vi "Move Set on Cursor Move.vi"(8 "Cursor.Position.X":dbl, 9 "Cursor Name":string, 10 "Refnums for Resizing and Alignment":T1, 11 "Display State In":T2={"Graph Visible Items"={"Plot Legend"=FALSE, "Scale Legend"=FALSE, "Graph Palette"=FALSE, "Cursor Legend"=FALSE, "X Scrollbar"=FALSE}, "View Table"=FALSE, "Table Visible Items"={"Vertical Scrollbar"=FALSE, "Horizontal Scrollbar"=FALSE, "Row Headers"=FALSE, "Column Headers"=FALSE, "Vertical Lines"=FALSE, "Horizontal Lines"=FALSE}, "Header Font"={"Font Name"="", "Size"=0, "Bold"=FALSE, "Italic"=FALSE, "Underline"=FALSE, "Strikeout"=FALSE, "Color"=0}, "Cell Font"={"Font Name"="", "Size"=0, "Bold"=FALSE, "Italic"=FALSE, "Underline"=FALSE, "Strikeout"=FALSE, "Color"=0}, "Description and Tip..."={"Description"="", "Tip"=""}, "Moveable Splitter Position"=0, "Measurement Cursor Configuration"={"relative to t0"={"enable relative time"=FALSE, "Relative times (DT)"=[], "color"=0}, "range"={"enable range"=FALSE, "T1"=0.0, "T2"=0.0, "Fixed interval (T2-T1)"=0.0, "T1 color"=0, "T2 color"=0, "enable shading"=FALSE}, "periodic"={"enable periodic"=FALSE, "First event (E1)"=0.0, "Number events (Ei)"=0, "Event spacing (s)"=0.0, "First color"=0, "Events color"=0}, "absolute timestamp"={"enable absolute"=FALSE, "Timestamps (TS)"=[], "color"=0}}, "X Increment"=0.0, "X Scale"={"Label Visible"=FALSE, "Label Text"="", "Time Mode"=enum."Relative", "Format String"=""}, "Y Scale"={"Label Visible"=FALSE, "Label Text"="", "Scaling"=enum."Engineering Units", "Format String"=""}, "Colors"={"background"=16777215, "major grid"=8355711, "minor grid"=12632256, "font"=0}, "Cursors"={"List"=[], "Tags"=[]}, "Plots"=[], "Plot Color Wheel"=[3381759, 32768, 982784, 4375295, 13827953, 13457919, 16757522, 4343295, 16728758, 12095254], "registered user events"=variant} caption="State") -> (1 "state changed":bool, 3 "Display State Out":T2={"Graph Visible Items"={"Plot Legend"=FALSE, "Scale Legend"=FALSE, "Graph Palette"=FALSE, "Cursor Legend"=FALSE, "X Scrollbar"=FALSE}, "View Table"=FALSE, "Table Visible Items"={"Vertical Scrollbar"=FALSE, "Horizontal Scrollbar"=FALSE, "Row Headers"=FALSE, "Column Headers"=FALSE, "Vertical Lines"=FALSE, "Horizontal Lines"=FALSE}, "Header Font"={"Font Name"="", "Size"=0, "Bold"=FALSE, "Italic"=FALSE, "Underline"=FALSE, "Strikeout"=FALSE, "Color"=0}, "Cell Font"={"Font Name"="", "Size"=0, "Bold"=FALSE, "Italic"=FALSE, "Underline"=FALSE, "Strikeout"=FALSE, "Color"=0}, "Description and Tip..."={"Description"="", "Tip"=""}, "Moveable Splitter Position"=0, "Measurement Cursor Configuration"={"relative to t0"={"enable relative time"=FALSE, "Relative times (DT)"=[], "color"=0}, "range"={"enable range"=FALSE, "T1"=0.0, "T2"=0.0, "Fixed interval (T2-T1)"=0.0, "T1 color"=0, "T2 color"=0, "enable shading"=FALSE}, "periodic"={"enable periodic"=FALSE, "First event (E1)"=0.0, "Number events (Ei)"=0, "Event spacing (s)"=0.0, "First color"=0, "Events color"=0}, "absolute timestamp"={"enable absolute"=FALSE, "Timestamps (TS)"=[], "color"=0}}, "X Increment"=0.0, "X Scale"={"Label Visible"=FALSE, "Label Text"="", "Time Mode"=enum."Relative", "Format String"=""}, "Y Scale"={"Label Visible"=FALSE, "Label Text"="", "Scaling"=enum."Engineering Units", "Format String"=""}, "Colors"={"background"=16777215, "major grid"=8355711, "minor grid"=12632256, "font"=0}, "Cursors"={"List"=[], "Tags"=[]}, "Plots"=[], "Plot Color Wheel"=[3381759, 32768, 982784, 4375295, 13827953, 13457919, 16757522, 4343295, 16728758, 12095254], "registered user events"=variant} caption="State")   [LabVIEW 2017, in "Waveforms with Cursors.xctl"]
doc: "Moves linked cursors in set. Also sets cursor selection in cursor table."
uses:
  <vilib>/addons/_XControls/Waveforms with Cursors/Waveforms with Cursors.xctl
  <vilib>/addons/_XControls/Waveforms with Cursors/Controls/State.ctl
  <vilib>/Utility/miscctls.llb/LVFontTypeDef.ctl
  <vilib>/addons/_XControls/Waveforms with Cursors/Controls/Waveform Cursor Configuration.ctl
  <vilib>/addons/_XControls/Waveforms with Cursors/Controls/Refnums Typedef.ctl
  <vilib>/Utility/miscctls.llb/LVRowAndColumnTypeDef.ctl
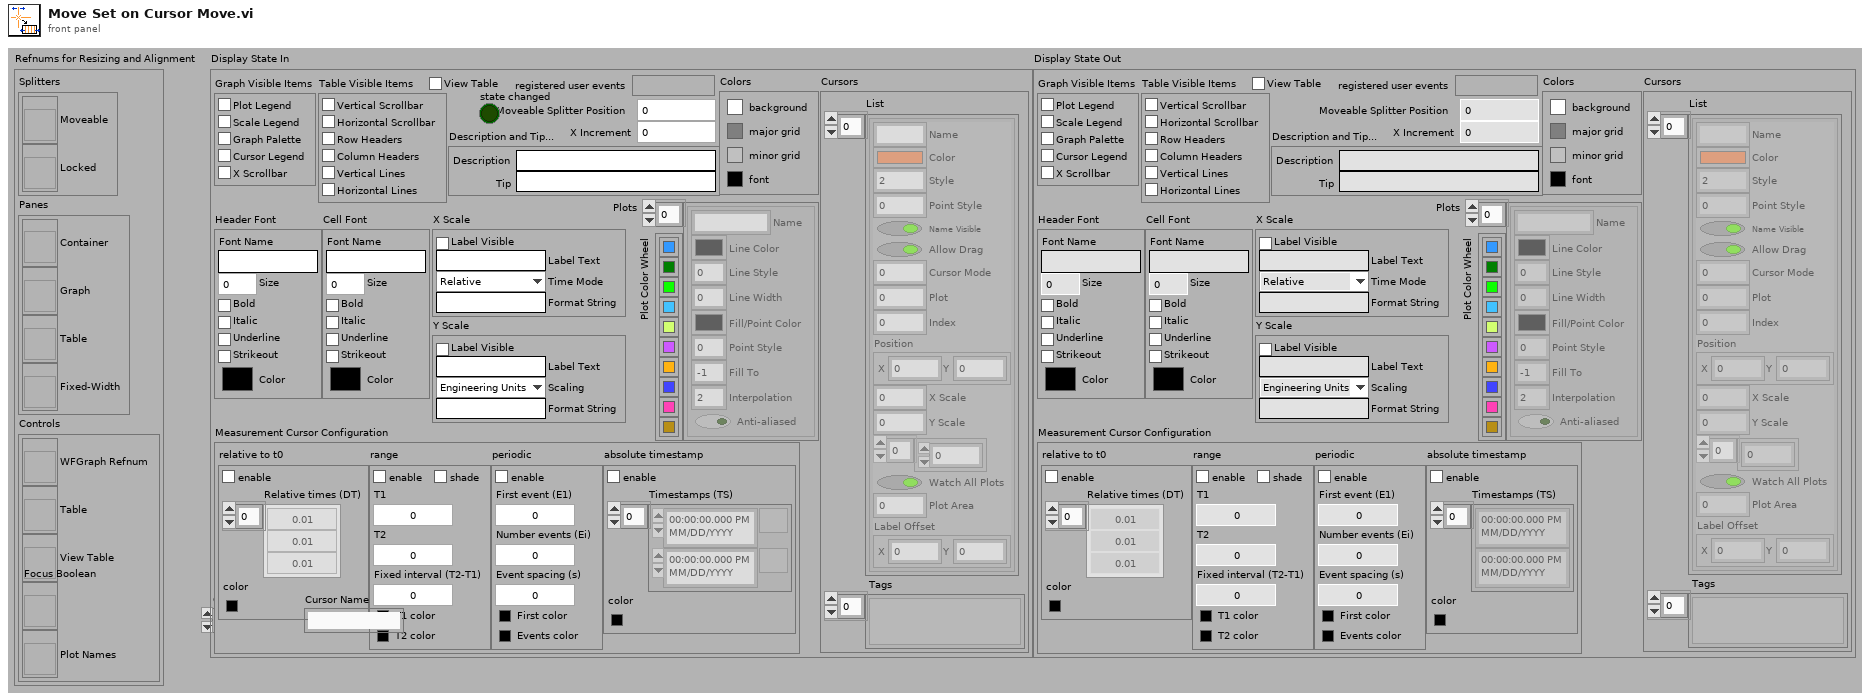
[diagram p1: front panel]
types:
  T1 = typedef "Waveforms with Cursors.xctl/Refnums Typedef.ctl" = cluster{"Splitters":cluster{"Moveable":refnum<vi>, "Locked":refnum<vi>}, "Panes":cluster{"Container":refnum<vi>, "Graph":refnum<vi>, "Table":refnum<vi>, "Fixed-Width":refnum<vi>}, "Controls":cluster{"WFGraph Refnum":refnum<vi>, "Table":refnum<vi>, "View Table":refnum<vi>, "Focus Boolean":refnum<vi>, "Plot Names":refnum<vi>}}
  T2 = typedef "Waveforms with Cursors.xctl/State.ctl" = cluster{"Graph Visible Items":cluster{"Plot Legend":bool, "Scale Legend":bool, "Graph Palette":bool, "Cursor Legend":bool, "X Scrollbar":bool}, "View Table":bool, "Table Visible Items":cluster{"Vertical Scrollbar":bool, "Horizontal Scrollbar":bool, "Row Headers":bool, "Column Headers":bool, "Vertical Lines":bool, "Horizontal Lines":bool}, "Header Font":T3, "Cell Font":T3, "Description and Tip...":cluster{"Description":string, "Tip":string}, "Moveable Splitter Position":i32, "Measurement Cursor Configuration":T4, "X Increment":dbl, "X Scale":cluster{"Label Visible":bool, "Label Text":string, "Time Mode":enum16{"Relative", "Absolute"}, "Format String":string}, "Y Scale":cluster{"Label Visible":bool, "Label Text":string, "Scaling":enum16{"Engineering Units", "Voltage"}, "Format String":string}, "Colors":cluster{"background":u32, "major grid":u32, "minor grid":u32, "font":u32}, "Cursors":cluster{"List":cluster{"Name":string, "Color":u32, "Style":i32, "Point Style":u8, "Name Visible":bool, "Allow Drag":bool, "Cursor Mode":u32, "Plot":i32, "Index":i32, "Position":cluster{"X":dbl, "Y":dbl}, "X Scale":u32, "Y Scale":u32, "Watch Plots":i32[], "Watch All Plots":bool, "Plot Area":i32, "Label Offset":cluster{"X":dbl, "Y":dbl}}[], "Tags":variant[]}, "Plots":cluster{"Name":string, "Line Color":u32, "Line Style":u8, "Line Width":u8, "Fill/Point Color":u32, "Point Style":u8, "Fill To":i16, "Interpolation":u8, "Anti-aliased":bool}[], "Plot Color Wheel":u32[], "registered user events":variant}
  T3 = typedef "LVFontTypeDef.ctl" = cluster{"Font Name":string, "Size":u16, "Bold":bool, "Italic":bool, "Underline":bool, "Strikeout":bool, "Color":u32}
  T4 = typedef "Waveforms with Cursors.xctl/Waveform Cursor Configuration.ctl" = cluster{"relative to t0":cluster{"enable relative time":bool, "Relative times (DT)":dbl[], "color":u32}, "range":cluster{"enable range":bool, "T1":dbl, "T2":dbl, "Fixed interval (T2-T1)":dbl, "T1 color":u32, "T2 color":u32, "enable shading":bool}, "periodic":cluster{"enable periodic":bool, "First event (E1)":dbl, "Number events (Ei)":i32, "Event spacing (s)":dbl, "First color":u32, "Events color":u32}, "absolute timestamp":cluster{"enable absolute":bool, "Timestamps (TS)":timestamp[], "color":u32}}
  T5 = cluster{"Name":string, "Color":u32, "Style":i32, "Point Style":u8, "Name Visible":bool, "Allow Drag":bool, "Cursor Mode":u32, "Plot":i32, "Index":i32, "Position":cluster{"X":dbl, "Y":dbl}, "X Scale":u32, "Y Scale":u32, "Watch Plots":i32[], "Watch All Plots":bool, "Plot Area":i32, "Label Offset":cluster{"X":dbl, "Y":dbl}}[]
  T6 = typedef "LVRowAndColumnTypeDef.ctl" = cluster{"Row":i32, "Column":i32}
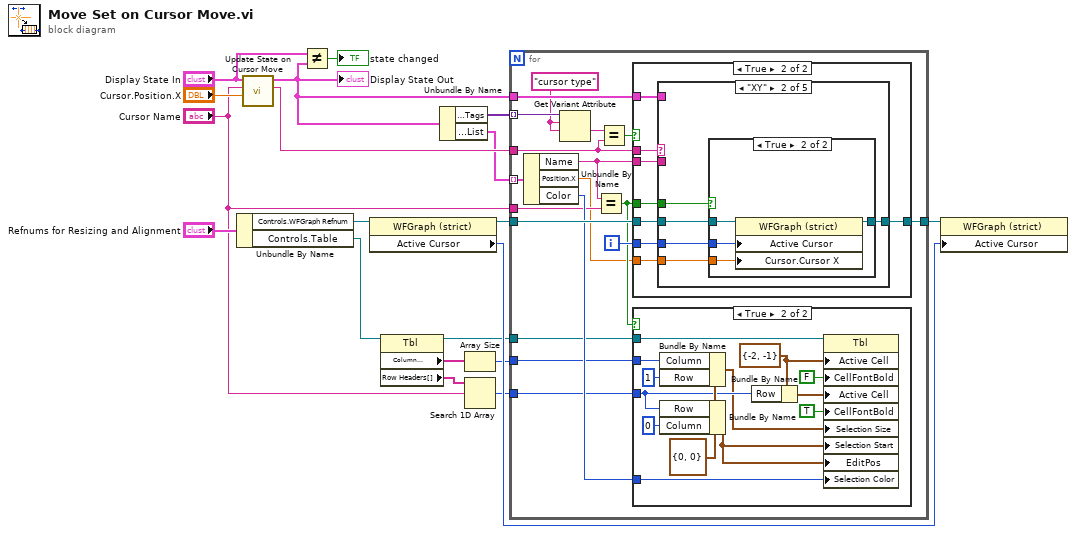
[diagram p0: block diagram]
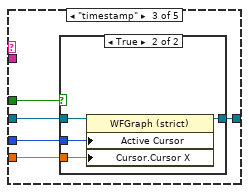
[diagram p6: hidden frame]
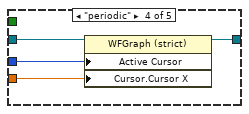
[diagram p8: hidden frame]
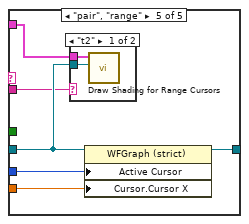
[diagram p9: hidden frame]
diagram:
  n1 = Unbundle By Name("Refnums for Resizing and Alignment") -> ("Controls.WFGraph Refnum"=w14:refnum<vi>, "Controls.Table"=w2:refnum<vi>)
  n2 = call <vilib>:"Update State on Cursor Move.vi"("Cursor.Position.X"="Cursor.Position.X", "Cursor Name"="Cursor Name", "Display State In"="Display State In") -> ("cursor type"=w12:string, "Display State out"=w10:T2)  [unwired: 7 in]
  "Display State Out" <- w10
  n3 = Not Equal?(x="Display State In", y=w10) -> (x != y?=→"state changed":bool)
  n4 = property class="WFGraph (strict)"(reference=w14) -> (reference out=w15:refnum<vi>, "Active Cursor"=w16:u32)  [unwired: 1 in, 1 out]
  n5 = property class="Tbl"(reference=w2) -> (reference out=w1:refnum<vi>, "Column Headers[]"=w6:string[], "Row Headers[]"=w7:string[])  [unwired: 1 in, 1 out]
  n6 = Unbundle By Name(w10) -> ("Cursors.Tags"=w11:variant[], "Cursors.List"=w8:T5)
  n7 = Array Size(array=w6) -> (size(s)=w5:i32)
  n8 = Search 1D Array(1D array=w7, element="Cursor Name") -> (index of element=w3:i32)  [unwired: 1 in]
  n9 = for {
    tunnel: w12 -> [w35]
    tunnel: w15 -> [w33]
    tunnel: "Cursor Name" -> [w24]
    tunnel: [w30] -> w13
    tunnel: w10 -> [w31]
    tunnel: w11 -> [w29] mode=indexing
    tunnel: w8 -> [w28] mode=indexing
    tunnel: w1 -> [w23]
    tunnel: w5 -> [w22]
    tunnel: w3 -> [w21]
    i -> [w32]
    w27 = "cursor type"
    n10 = Unbundle By Name(w28) -> ("Name"=w34:string, "Position.X"=w20:dbl, "Color"=w26:u32)
    n11 = Get Variant Attribute(Variant=w29, name=w27, default value (empty Variant)=w27) -> (value=w36:string)  [unwired: 1 in, 3 out]
    n12 = Equal?(x=w34, y=w24) -> (x = y?=w25:bool)
    n13 = Equal?(x=w36, y=w35) -> (x = y?=w37:bool)
    n14 = case shown="True" w37 {
      tunnel: w31 -> [_ w59]
      tunnel: w35 -> [_ w58]
      tunnel: w33 -> [w51 w57]
      tunnel: w25 -> [_ w54]
      tunnel: w34 -> [_ w56]
      tunnel: w32 -> [_ w55]
      tunnel: [w51 w53] -> w30
      tunnel: w20 -> [_ w52]
      frame False {
      }
      frame True {
        n15 = case shown="\"XY\"" w58 {
          tunnel: w59 -> [_ _ _ _ w88]
          tunnel: w57 -> [w60 w65 w75 w83 w87]
          tunnel: w56 -> [_ _ _ _ w85]
          tunnel: w55 -> [_ w64 w74 w84 w90]
          tunnel: w54 -> [_ w63 w73 _ _]
          tunnel: [w60 w62 w72 w82 w89] -> w53
          tunnel: w52 -> [_ w61 w71 w81 w86]
          frame Default {
          }
          frame "XY" {
            n16 = case shown="True" w63 {
              tunnel: w65 -> [w66 w70]
              tunnel: w61 -> [_ w69]
              tunnel: w64 -> [_ w68]
              tunnel: [w66 w67] -> w62
              frame False {
              }
              frame True {
                n17 = property class="WFGraph (strict)"(reference=w70, "Active Cursor"=w68, "Cursor.Cursor X"=w69) -> (reference out=w67:refnum<vi>)  [unwired: 1 in, 1 out]
              }
            }
          }
          frame "timestamp" {
            n18 = case shown="True" w73 {
              tunnel: w75 -> [w76 w80]
              tunnel: w71 -> [_ w79]
              tunnel: w74 -> [_ w78]
              tunnel: [w76 w77] -> w72
              frame False {
              }
              frame True {
                n19 = property class="WFGraph (strict)"(reference=w80, "Active Cursor"=w78, "Cursor.Cursor X"=w79) -> (reference out=w77:refnum<vi>)  [unwired: 1 in, 1 out]
              }
            }
          }
          frame "periodic" {
            n20 = property class="WFGraph (strict)"(reference=w83, "Active Cursor"=w84, "Cursor.Cursor X"=w81) -> (reference out=w82:refnum<vi>)  [unwired: 1 in, 1 out]
          }
          frame "pair", "range" {
            n21 = case shown="\"t2\"" w85 {
              tunnel: w88 -> [w92 _]
              tunnel: w87 -> [w91 _]
              frame "t2" {
                n22 = call <vilib>:"Draw Shading for Range Cursors.vi"("WaveformGraph"=w91, "Display State In"=w92) -> ()  [unwired: 9 in, 1 out]
              }
              frame Default {
              }
            }
            n23 = property class="WFGraph (strict)"(reference=w87, "Active Cursor"=w90, "Cursor.Cursor X"=w86) -> (reference out=w89:refnum<vi>)  [unwired: 1 in, 1 out]
          }
        }
      }
    }
    n24 = case shown="True" w25 {
      tunnel: w23 -> [_ w44]
      tunnel: w26 -> [_ w40]
      tunnel: w22 -> [_ w38]
      tunnel: w21 -> [_ w43]
      frame False {
      }
      frame True {
        w48 = T6 {"Row"=-2, "Column"=-1} ("Active Cell:Active Cell")
        w46 = T6 {"Row"=0, "Column"=0} ("Selection Size")
        n25 = Bundle By Name(cluster=w46, "Column"=w38, "Row"=1) -> (w42:T6)
        n26 = Bundle By Name(cluster=w46, "Row"=w43, "Column"=0) -> (w41:T6)
        n27 = Bundle By Name(cluster=w48, "Row"=w43) -> (w47:T6)
        n28 = property class="Tbl"(reference=w44, "Active Cell"=w48, "CellFontBold"=FALSE ("Active Cell:Cell Font:Bold"), "Active Cell"=w47, "CellFontBold"=TRUE ("Active Cell:Cell Font:Bold"), "Selection Size"=w42, "Selection Start"=w41, "EditPos"=w41, "Selection Color"=w40) -> ()  [unwired: 1 in, 2 out]
      }
    }
  }
  n29 = property class="WFGraph (strict)"(reference=w13, "Active Cursor"=w16) -> ()  [unwired: 1 in, 2 out]
